vi "Quick stop.vi"(8 "Fehler (Eingang, kein Fehler)":errorcluster) -> (0 "error out":errorcluster)   [LabVIEW 2014]
uses:
  <vilib>/CANopenLib/CANOPEN.llb/CANopen SDO Create.vi
  <vilib>/CANopenLib/CANOPEN.llb/CANopen SDO Write [U16].vi
  <vilib>/CANopenLib/CANOPEN.llb/CANopen SDO Close.vi
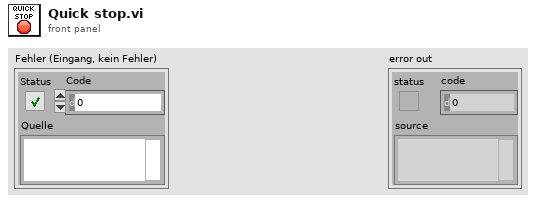
[diagram p1: front panel]
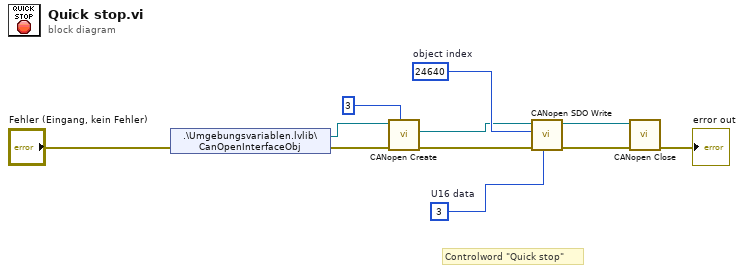
[diagram p0: block diagram]
diagram:
  w4 = u16 3  # U16 data
  w10 = u16 24640  # object index
  # "Controlword \"Quick stop\""
  n1 = shared-variable ".\\Umgebungsvariablen.lvlib\\CanOpenInterfaceObj"(error in="Fehler (Eingang, kein Fehler)") -> (w9:refnum<k20>, error out=w8:errorcluster)
  n2 = call-poly <vilib>:"CANopen Create.vi"("node-ID"=u8 3, "error in (no error)"=w8, "interface object in"=w9) -> ("error out"=w5:errorcluster, "SDO object out"=w6:refnum<k20>)  [unwired: 6 in, 1 out]
  n3 = call-poly <vilib>:"CANopen SDO Write.vi"("U16 data"=w4, "error in (no error)"=w5, "object index"=w10, "SDO object in"=w6) -> ("error out"=w3:errorcluster, "SDO object out"=w2:refnum<k20>)  [unwired: 5 in, 1 out]
  n4 = call-poly <vilib>:"CANopen Close.vi"("error in (no error)"=w3, "SDO object in"=w2) -> ("error out"=→"error out":errorcluster)  [unwired: 9 in]
